vi "_check_V.vi"(1 "输入":i8[](array[numeric])) -> (0 "输出":i8[](array[numeric]))   [LabVIEW 2018]
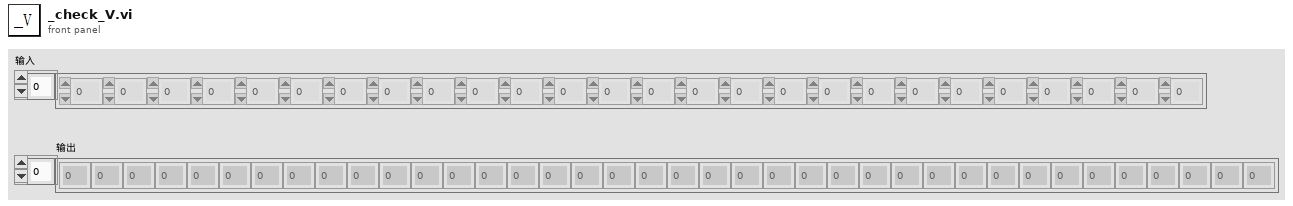
[diagram p1: front panel]
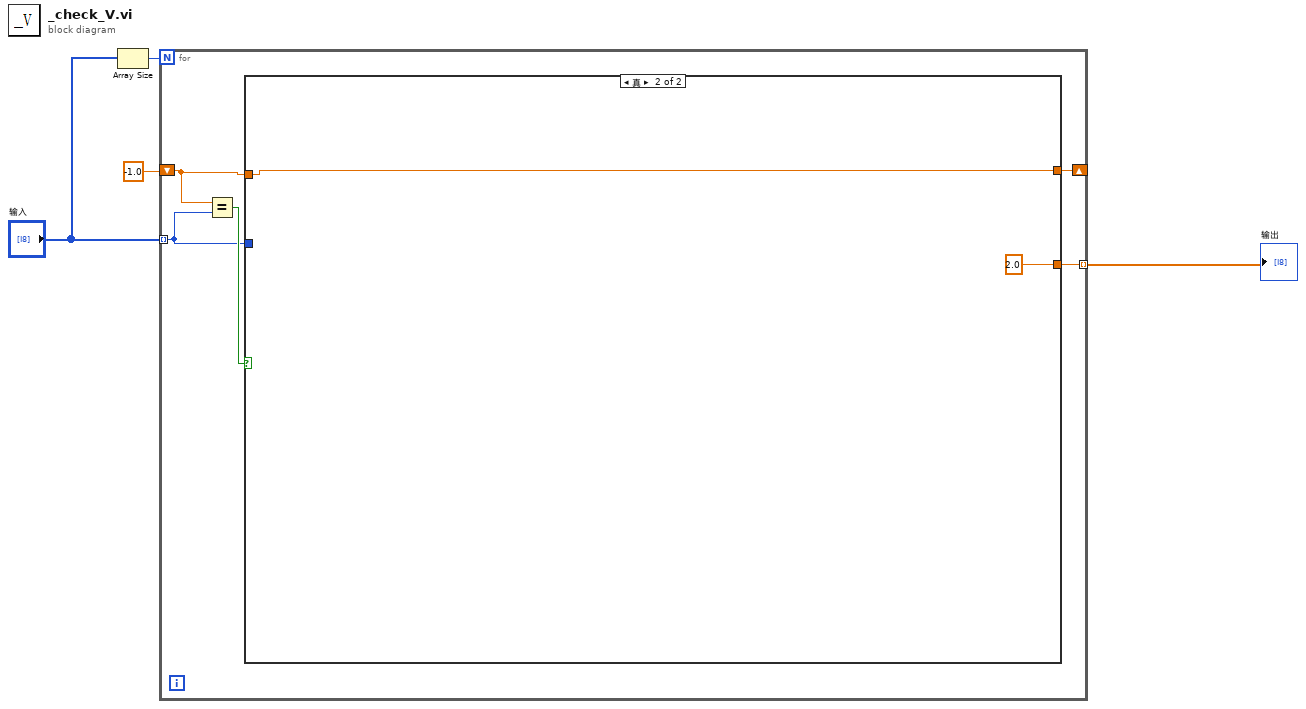
[diagram p0: block diagram]
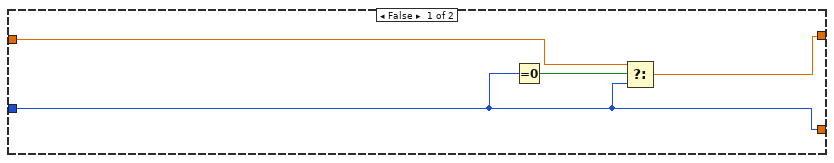
[diagram p2: hidden frame]
diagram:
  n1 = Array Size(array="输入") -> (size(s)=w4:i32)
  n2 = for {
    N: w4 -> [_]
    tunnel: "输入" -> [w5] mode=indexing
    shift-right: [w6] -> _
    shift-left: -1.0 -> [w7]
    tunnel: [w8] -> w1 mode=indexing
    n3 = Equal?(x=w7, y=w5) -> (x = y?=w9:bool)
    n4 = case shown="真" w9 {
      tunnel: [w10 2.0] -> w8
      tunnel: w7 -> [w12 w14]
      tunnel: [w11 w14] -> w6
      tunnel: w5 -> [w10 _]
      frame False {
        n5 = Equal To 0?(x=w10) -> (x = 0?=w13:bool)
        n6 = Select(t=w12, s=w13, f=w10) -> (s? t:f=w11:dbl)
      }
      frame True {
      }
    }
  }
  "输出" <- w1
